vi "programa5.vi"() -> ()   [LabVIEW 2011]
panel:
  out "Personas":dbl
  in  "Planta":u16(ring) items=["Planta #1", "Planta #2", "Planta #3"]
  out "Aire Acondicionado":bool
  out "Temperatura":i32(slide) scale=0.0..60.0
  # "Se genera la temperatura entre 1-60,\nse selecciona la planta usando el menu ring, \nluego se gerena el numero de personas entre 1-50"
  # "Planta 1 si hay mas de 25 personas y las temperatura \nes mayor a 22 se enciende el A/C\n\nPlanta 2 si hay mas de 30 personas y las temperatura \nes mayor a 27 se enciende el A/C\n\nPlanta 3 si hay mas de 20 personas y las temperatura \nes mayor a 29 se enciende el A/C"
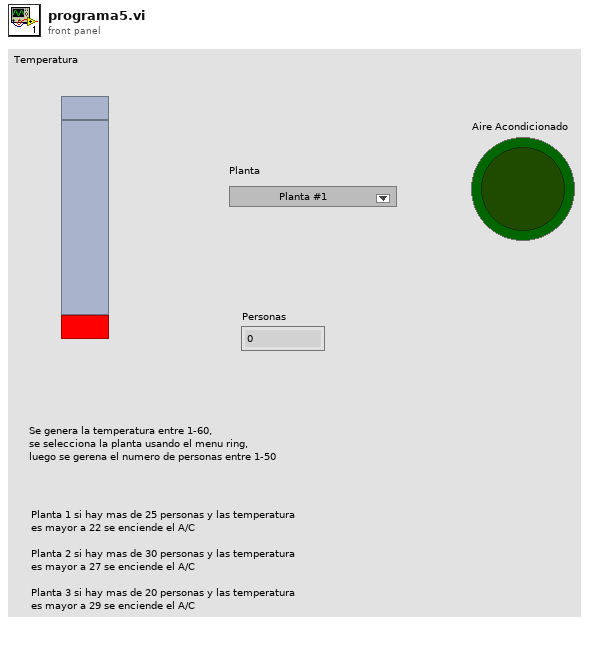
[diagram p1: front panel]
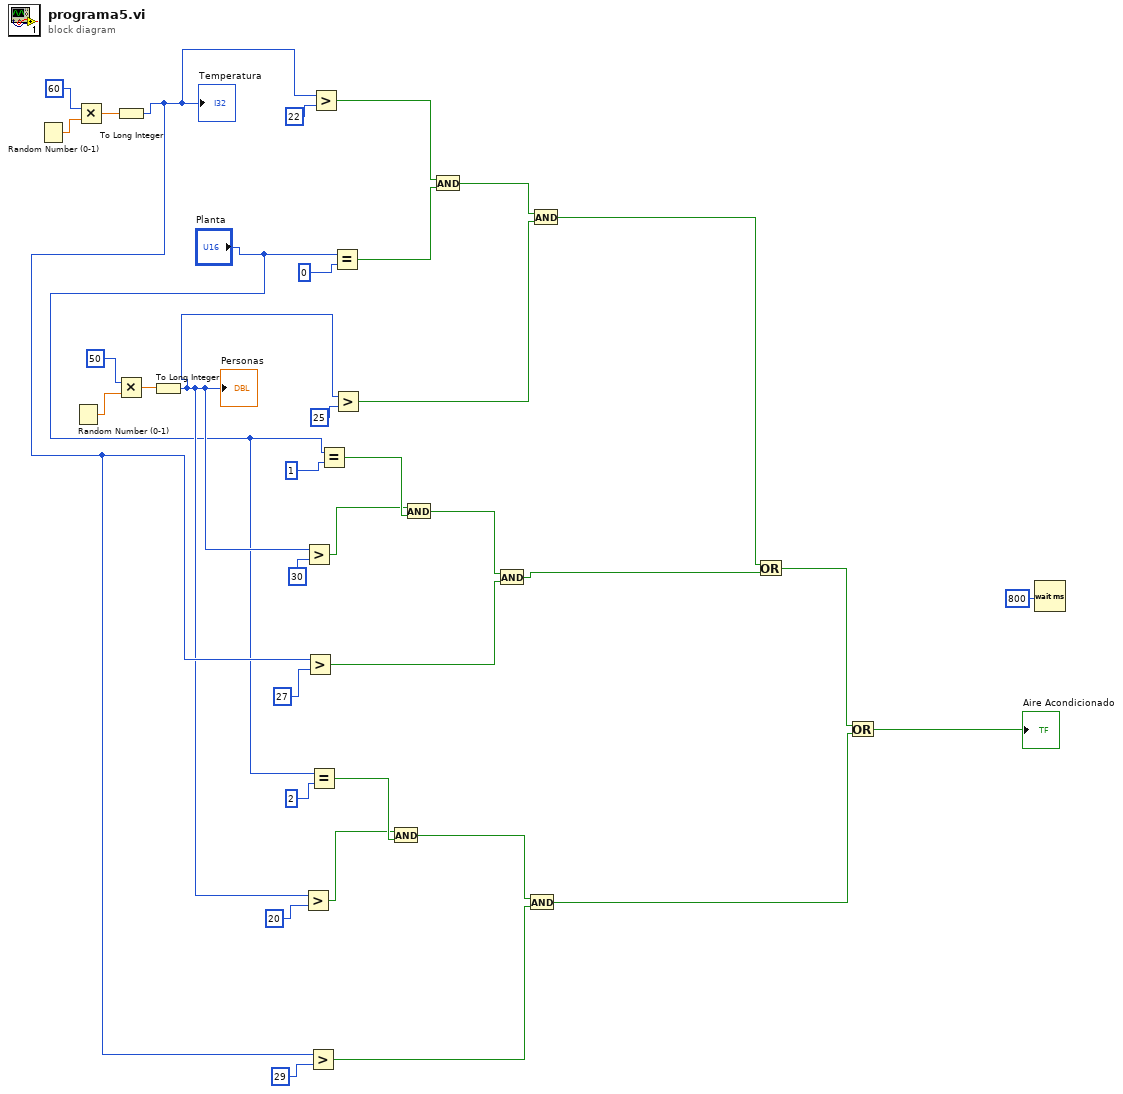
[diagram p0: block diagram]
diagram:
  n1 = Random Number (0-1)() -> (number: 0 to 1=w35:dbl)
  n2 = Random Number (0-1)() -> (number: 0 to 1=w33:dbl)
  n3 = Multiply(x=60, y=w35) -> (x*y=w34:dbl)
  n4 = To Long Integer(number=w34) -> (32bit integer=w15:i32)
  "Temperatura" <- w15
  n5 = Multiply(x=50, y=w33) -> (x*y=w32:dbl)
  n6 = To Long Integer(number=w32) -> (32bit integer=w14:i32)
  "Personas" <- w14
  n7 = Greater?(x=w14, y=20) -> (0:w10:bool)
  n8 = Greater?(x=w14, y=30) -> (0:w20:bool)
  n9 = Greater?(x=w15, y=27) -> (0:w18:bool)
  n10 = Greater?(x=w15, y=29) -> (0:w8:bool)
  n11 = Equal?(x="Planta", y=2) -> (x = y?=w11:bool)
  n12 = Greater?(x=w15, y=22) -> (0:w27:bool)
  n13 = Equal?(x="Planta", y=1) -> (x = y?=w21:bool)
  n14 = Equal?(x="Planta", y=0) -> (x = y?=w26:bool)
  n15 = Greater?(x=w14, y=25) -> (0:w24:bool)
  n16 = And(x=w10, y=w11) -> (x .and. y?=w9:bool)
  n17 = And(x=w20, y=w21) -> (x .and. y?=w19:bool)
  n18 = And(x=w27, y=w26) -> (x .and. y?=w25:bool)
  n19 = And(x=w19, y=w18) -> (x .and. y?=w6:bool)
  n20 = And(x=w9, y=w8) -> (x .and. y?=w4:bool)
  n21 = And(x=w25, y=w24) -> (x .and. y?=w7:bool)
  n22 = Or(x=w7, y=w6) -> (x .or. y?=w5:bool)
  n23 = Or(x=w5, y=w4) -> (x .or. y?=→"Aire Acondicionado":bool)
  n24 = Wait (ms)(milliseconds to wait=800) -> ()  [unwired: 1 out]
